vi "FGV Schedule Log.vi"(0 "Neuer Eintrag":string, 11 "error in (no error)":errorcluster caption="Fehler (Eingang, kein Fehler)", 13 "Aktion":T1) -> (4 "Anzeige":string[](array[string]), 8 "Log Array":string[](array[string]), 10 "Fehler":bool[](array[boolean]), 15 "error out":errorcluster caption="Fehler (Ausgang)")   [LabVIEW 2015, in "Schedule Modul.lvlib"]
uses:
  Schedule Modul.lvlib
  Aktion FGV Schedule Log.ctl
  Allgemein/allgemeine Sub-VIs.lvlib
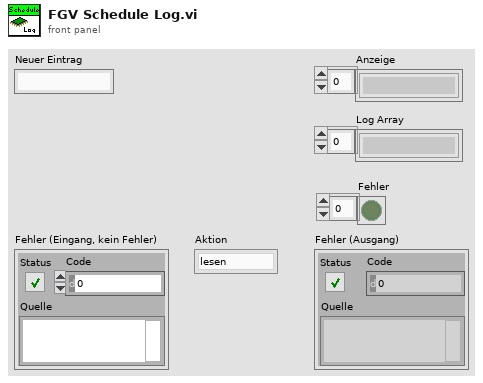
[diagram p1: front panel]
types:
  T1 = typedef "Schedule Modul.lvlib/Aktion FGV Schedule Log.ctl" = enum16{"lesen", "neuer Eintrag", "laden", "löschen", "Anzeige löschen"}
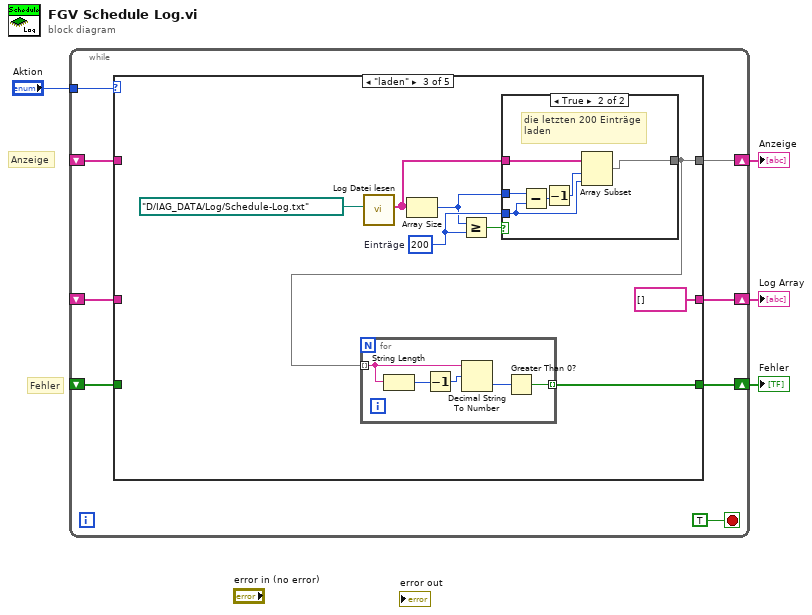
[diagram p0: block diagram]
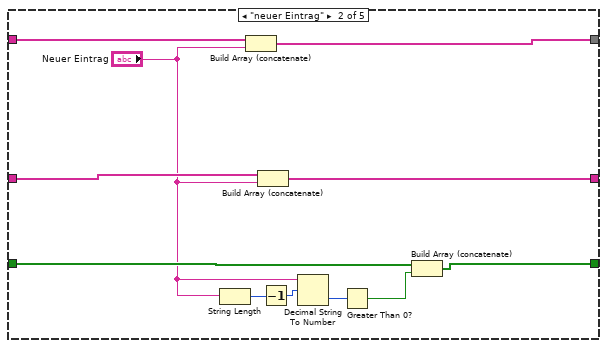
[diagram p3: hidden frame]
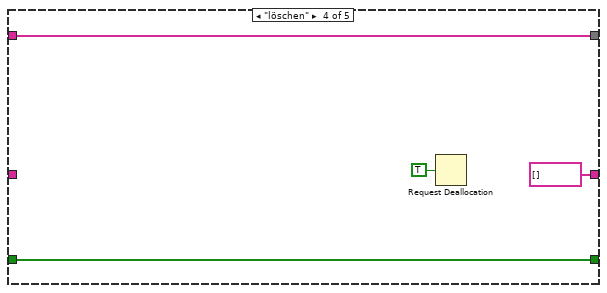
[diagram p5: hidden frame]
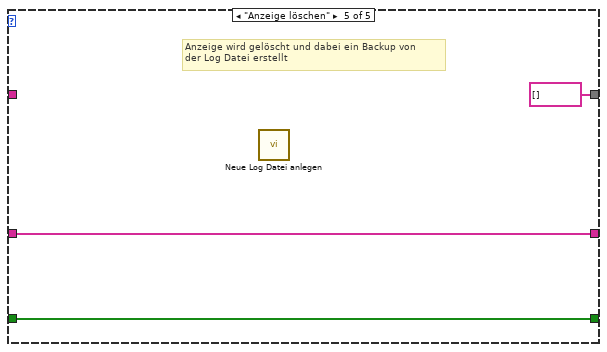
[diagram p6: hidden frame]
diagram:
  # "Fehler"
  # "Anzeige"
  n1 = while {
    tunnel: "Aktion" -> [w11]
    shift-right: [w10] -> w3
    shift-left: _ -> [w9]
    shift-right: [w8] -> w2
    shift-left: _ -> [w7]
    shift-right: [w6] -> w1
    shift-left: _ -> [w5]
    stop <- TRUE stop-if-true
    n2 = case shown="\"laden\"" w11 {
      tunnel: [w15 w26 w28 w49 string[] [] ("Array")] -> w10
      tunnel: w9 -> [w15 w25 _ w49 _]
      tunnel: [w14 w24 string[] [] string[] [] w53] -> w8
      tunnel: w7 -> [w14 w23 _ _ w53]
      tunnel: [w13 w21 w27 w47 w51] -> w6
      tunnel: w5 -> [w13 w22 _ w47 w51]
      frame "lesen", Default {
      }
      frame "neuer Eintrag" {
        n3 = String Length(string="Neuer Eintrag") -> (length=w20:i32)
        n4 = Build Array (concatenate)(w25, "Neuer Eintrag") -> (w26:string[])
        n5 = Build Array (concatenate)(w23, "Neuer Eintrag") -> (w24:string[])
        n6 = Decrement(x=w20) -> (x-1=w19:i32)
        n7 = Decimal String To Number(string="Neuer Eintrag", offset=w19) -> (number=w18:i32)  [unwired: 1 in, 1 out]
        n8 = Greater Than 0?(x=w18) -> (x > 0?=w17:bool)
        n9 = Build Array (concatenate)(w22, w17) -> (w21:bool[])
      }
      frame "laden" {
        w31 = 200  # Einträge
        n10 = call "Log Datei lesen.vi"("Dateipfad"=path "D:/IAG_DATA/Log/Schedule-Log.txt" ("Datei")) -> ("Array"=w32:string[])  [unwired: 10 in]
        n11 = Array Size(array=w32) -> (size(s)=w29:i32)
        n12 = Greater Or Equal?(x=w29, y=w31) -> (x >= y?=w33:bool)
        n13 = case shown="True" w33 {
          tunnel: [w40 w41] -> w28
          tunnel: w32 -> [w40 w46]
          tunnel: w31 -> [_ w43]
          tunnel: w29 -> [_ w45]
          frame False {
          }
          frame True {
            # "die letzten 200 Einträge\nladen"
            n14 = Subtract(x=w45, y=w43) -> (x-y=w44:i32)
            n15 = Decrement(x=w44) -> (x-1=w42:i32)
            n16 = Array Subset(array=w46, index=w42, length=w43) -> (w41:string[])
          }
        }
        n17 = for {
          tunnel: w28 -> [w38] mode=indexing
          tunnel: [w35] -> w27 mode=indexing
          n18 = String Length(string=w38) -> (length=w39:i32)
          n19 = Decrement(x=w39) -> (x-1=w37:i32)
          n20 = Decimal String To Number(string=w38, offset=w37) -> (number=w36:i32)  [unwired: 1 in, 1 out]
          n21 = Greater Than 0?(x=w36) -> (x > 0?=w35:bool)
        }
      }
      frame "löschen" {
        n22 = Request Deallocation(TRUE ("Flag")) -> ()
      }
      frame "Anzeige löschen" {
        # "Anzeige wird gelöscht und dabei ein Backup von \nder Log Datei erstellt"
        n23 = call "Neue Log Datei anlegen.vi"() -> ()  [unwired: 11 in, 1 out]
      }
    }
  }
  "Anzeige" <- w3
  "Log Array" <- w2
  "Fehler" <- w1
